vi "MinimalCaptureExample.vi"() -> ()   [LabVIEW 2020]
uses:
  C:/Users/Public/Documents/Photometrics/TPM-LabVIEWSamples/Examples/2020/Dependencies/PVCamNET.dll
  Public/Documents/Photometrics/TPM-LabVIEWSamples/Examples/2020/Dependencies/PVCamNET.dll
  shell32.dll
panel:
  out "Image Data":u16[][](array[numeric])
  out "Error":errorcluster
  out "Current Frame":u32
  out "Sensor Width":u32
  out "Sensor Height":u32
  out "Camera Name":string
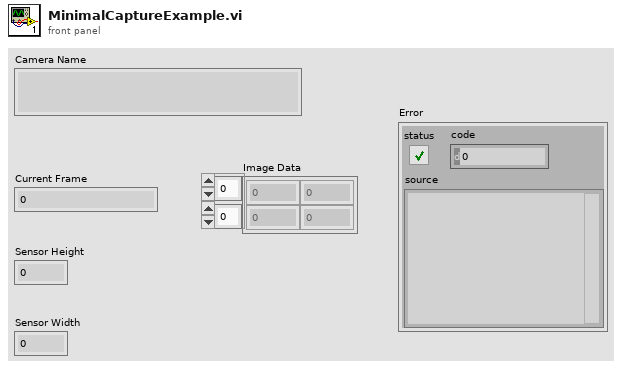
[diagram p1: front panel]
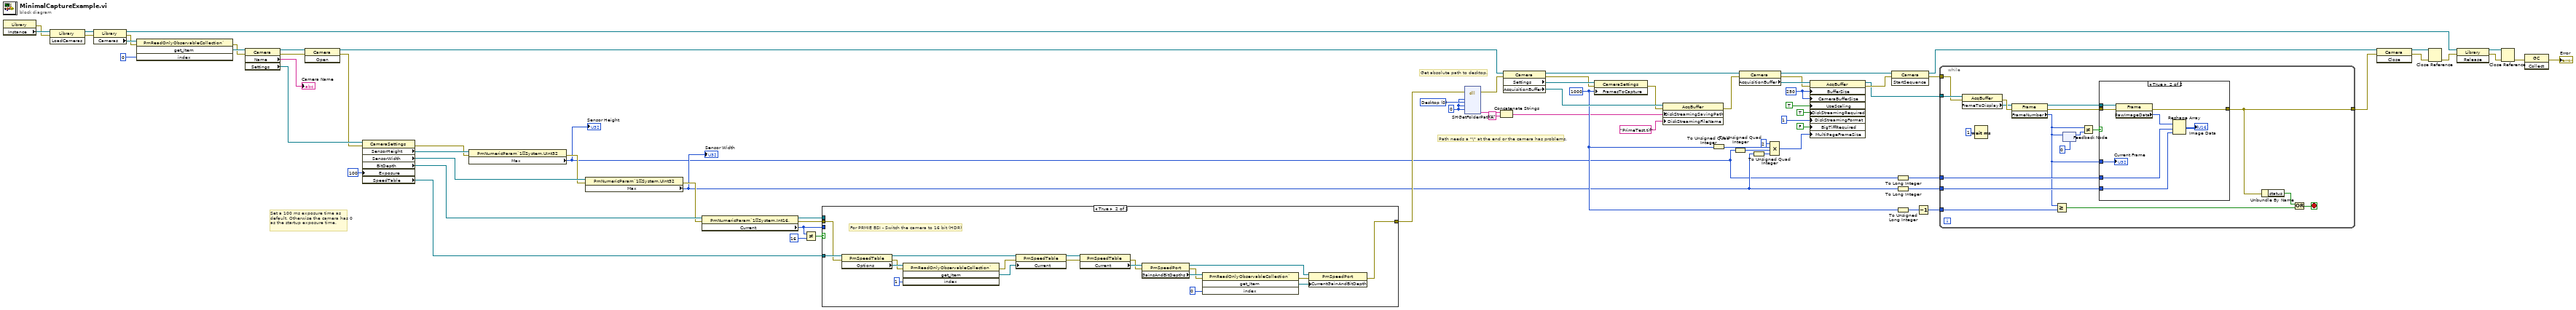
[diagram p0: block diagram]
diagram:
  w20 = u32 250 ("BufferSize")
  w11 = u16 1000 ("FramesToCapture")
  w41 = 0 items=["Desktop"=0, "Personal Documents"=5, "AppData"=26, "Local AppData"=28, "Common AppData"=35, "Program Files"=38, "Program Files Common"=43, "Common Documents"=46] ("Requested Path")
  w40 = 0 ("HWND")
  # "Path needs a \"\\\" at the end or the camera has problems."
  # "Get absolute path to desktop."
  # "Set a 100 ms exposure time as default. Otherwise the camera has 0 as the startup exposure time."
  n1 = property class="Library"() -> (error out=w72:errorcluster, "Instance"=w75:refnum<k24>)  [unwired: 2 in, 1 out]
  n2 = invoke class="Library" method="LoadCameras"(reference=w75, error in=w72) -> (reference out=w74:refnum<k24>, error out=w71:errorcluster)  [unwired: 1 in, 1 out]
  n3 = property class="Library"(reference=w74, error in=w71) -> (reference out=w60:refnum<k24>, error out=w70:errorcluster, "Cameras"=w73:refnum<k24>)
  n4 = invoke class="PmReadOnlyObservableCollection`" method="get_Item"(reference=w73, error in=w70, "index"=0) -> (error out=w68:errorcluster, "get_Item"=w69:refnum<k24>)  [unwired: 1 in, 2 out]
  n5 = property class="Camera"(reference=w69, error in=w68) -> (reference out=w66:refnum<k24>, error out=w58:errorcluster, "Name"=→"Camera Name":string, "Settings"=w67:refnum<k24>)
  n6 = invoke class="Camera" method="Open"(reference=w66, error in=w58) -> (reference out=w35:refnum<k24>, error out=w57:errorcluster)  [unwired: 1 in, 1 out]
  n7 = property class="CameraSettings"(reference=w67, error in=w57, "Exposure"=u32 100) -> (error out=w54:errorcluster, "SensorHeight"=w56:refnum<k24>, "SensorWidth"=w55:refnum<k24>, "BitDepth"=w52:refnum<k24>, "SpeedTable"=w49:refnum<k24>)  [unwired: 1 out]
  n8 = property class="PmNumericParam`1[[System.UInt32"(reference=w56, error in=w54) -> (error out=w53:errorcluster, "Max"=w3:u32)  [unwired: 1 out]
  "Sensor Height" <- w3
  n9 = property class="PmNumericParam`1[[System.UInt32"(reference=w55, error in=w53) -> (error out=w51:errorcluster, "Max"=w4:u32)  [unwired: 1 out]
  "Sensor Width" <- w4
  n10 = property class="PmNumericParam`1[[System.Int16,"(reference=w52, error in=w51) -> (reference out=w62:refnum<k24>, error out=w61:errorcluster, "Current"=w59:i16)
  n11 = Not Equal?(x=w59, y=i16 16) -> (x != y?=w63:bool)
  n12 = case shown="True" w63 {
    tunnel: w62 -> [_ _]
    tunnel: w61 -> [w76 w92]
    tunnel: [w76 w77] -> w33
    tunnel: w59 -> [_ _]
    tunnel: w49 -> [_ w95]
    frame False {
    }
    frame True {
      # "For PRMIE BSI - Switch the camera to 16 bit (HDR)"
      n13 = property class="PmSpeedTable"(reference=w95, error in=w92) -> (reference out=w90:refnum<k24>, error out=w91:errorcluster, "Options"=w94:refnum<k24>)
      n14 = invoke class="PmReadOnlyObservableCollection`" method="get_Item"(reference=w94, error in=w91, "index"=1) -> (error out=w89:errorcluster, "get_Item"=w88:refnum<k24>)  [unwired: 1 in, 2 out]
      n15 = property class="PmSpeedTable"(reference=w90, error in=w89, "Current"=w88) -> (reference out=w87:refnum<k24>, error out=w86:errorcluster)
      n16 = property class="PmSpeedTable"(reference=w87, error in=w86) -> (error out=w83:errorcluster, "Current"=w85:refnum<k24>)  [unwired: 1 out]
      n17 = property class="PmSpeedPort"(reference=w85, error in=w83) -> (reference out=w78:refnum<k24>, error out=w82:errorcluster, "GainsAndBitDepths"=w84:refnum<k24>)
      n18 = invoke class="PmReadOnlyObservableCollection`" method="get_Item"(reference=w84, error in=w82, "index"=0) -> (error out=w79:errorcluster, "get_Item"=w80:refnum<k24>)  [unwired: 1 in, 2 out]
      n19 = property class="PmSpeedPort"(reference=w78, error in=w79, "CurrentGainAndBitDepth"=w80) -> (error out=w77:errorcluster)  [unwired: 1 out]
    }
  }
  n20 = dll-call lib="shell32.dll" fn="SHGetFolderPathA"(error in=w33, "HWND"=w40, "nFolder"=w41, "hToken"=w40, "dwFlags"=w40) -> (error out=w32:errorcluster, "pszPath"=w7:string)  [unwired: 8 in, 1 out]
  n21 = Concatenate Strings(w7, "\\" ("string")) -> (w5:string)
  n22 = property class="Camera"(reference=w35, error in=w32) -> (reference out=w19:refnum<k24>, error out=w38:errorcluster, "Settings"=w39:refnum<k24>, "AcquisitionBuffer"=w37:refnum<k24>)
  n23 = property class="CameraSettings"(reference=w39, error in=w38, "FramesToCapture"=w11) -> (error out=w36:errorcluster)  [unwired: 1 out]
  n24 = property class="AcqBuffer"(reference=w37, error in=w36, "DiskStreamingSavingPath"=w5, "DiskStreamingFileName"="PrimeTest.tif") -> (error out=w18:errorcluster)  [unwired: 1 out]
  n25 = To Unsigned Quad Integer(1:w11) -> (0:w24:u64)
  n26 = To Unsigned Quad Integer(1:w3) -> (0:w22:u64)
  n27 = property class="Camera"(reference=w19, error in=w18) -> (reference out=w17:refnum<k24>, error out=w30:errorcluster, "AcquisitionBuffer"=w31:refnum<k24>)
  n28 = To Unsigned Quad Integer(1:w4) -> (0:w23:u64)
  n29 = Compound Arithmetic op=MULTIPLY(u64 2 ("value"), w24, w22, w23) -> (w21:u64)
  n30 = property class="AcqBuffer"(reference=w31, error in=w30, "BufferSize"=w20, "CameraBufferSize"=w20, "UseScaling"=TRUE, "DiskStreamingRequired"=TRUE, "DiskStreamingFormat"=u32 1, "BigTiffRequired"=FALSE, "MultiPageFrameSize"=w21) -> (reference out=w15:refnum<k24>, error out=w16:errorcluster)
  n31 = invoke class="Camera" method="StartSequence"(reference=w17, error in=w16) -> (reference out=w13:refnum<k24>, error out=w14:errorcluster)  [unwired: 1 in, 1 out]
  n32 = To Long Integer(number=w3) -> (32bit integer=w2:i32)
  n33 = To Long Integer(number=w4) -> (32bit integer=w1:i32)
  n34 = To Unsigned Long Integer(number=w11) -> (unsigned 32bit integer=w10:u32)
  n35 = Decrement(x=w10) -> (x-1=w12:u32)
  n36 = while {
    tunnel: w15 -> [w111]
    tunnel: w14 -> [w110]
    tunnel: w12 -> [w109]
    tunnel: [w96] -> w9
    tunnel: w1 -> [w99]
    tunnel: w2 -> [w100]
    stop <- w106 stop-if-true
    n37 = property class="AcqBuffer"(reference=w111, error in=w110) -> (error out=w113:errorcluster, "FrameToDisplay"=w112:refnum<k24>)  [unwired: 1 out]
    n38 = Wait (ms)(milliseconds to wait=u32 1) -> ()  [unwired: 1 out]
    n39 = property class="Frame"(reference=w112, error in=w113) -> (reference out=w101:refnum<k24>, error out=w98:errorcluster, "FrameNumber"=w97:u32)
    n40 = Greater Or Equal?(x=w97, y=w109) -> (x >= y?=w108:bool)
    n41 = feedback #1(u32 0 ("FrameNumber")) -> (w103:u32)
    n42 = feedback-in #1(w97) -> ()
    n43 = Not Equal?(x=w97, y=w103) -> (x != y?=w102:bool)
    n44 = case shown="True" w102 {
      tunnel: w101 -> [_ w122]
      tunnel: w100 -> [_ w121]
      tunnel: w99 -> [_ w120]
      tunnel: w98 -> [w114 w119]
      tunnel: [w114 w117] -> w96
      tunnel: w97 -> [_ w118]
      frame False {
      }
      frame True {
        n45 = property class="Frame"(reference=w122, error in=w119) -> (error out=w117:errorcluster, "RawImageData"=w115:u16[])  [unwired: 1 out]
        n46 = Reshape Array(w115, w121, w120) -> (→"Image Data":u16[][])
        "Current Frame" <- w118
      }
    }
    n47 = Unbundle By Name(w96) -> ("status"=w107:bool)
    n48 = Or(x=w107, y=w108) -> (x .or. y?=w106:bool)
  }
  n49 = invoke class="Camera" method="Close"(reference=w13, error in=w9) -> (reference out=w46:refnum<k24>, error out=w44:errorcluster)  [unwired: 1 in, 1 out]
  n50 = Close Reference(reference=w46, error in (no error)=w44) -> (error out=w43:errorcluster)
  n51 = invoke class="Library" method="Release"(reference=w60, error in=w43) -> (reference out=w45:refnum<k24>, error out=w48:errorcluster)  [unwired: 1 in, 1 out]
  n52 = Close Reference(reference=w45, error in (no error)=w48) -> (error out=w47:errorcluster)
  n53 = invoke class="GC" method="Collect"(error in=w47) -> (error out=→"Error":errorcluster)  [unwired: 2 in, 2 out]
